vi "Get Source Directories.vi"() -> (1 "Runtime Dir":path, 2 "Protos Dir":path, 3 "Source Dir":path)   [LabVIEW 2020]
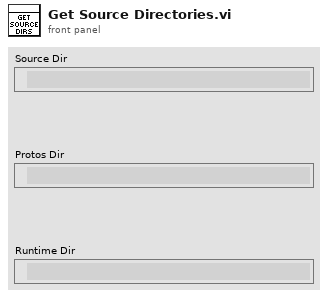
[diagram p1: front panel]
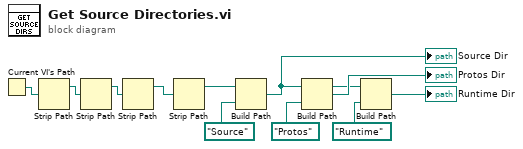
[diagram p0: block diagram]
diagram:
  n1 = Current VI's Path() -> (path=w8:path)
  n2 = Strip Path(path=w8) -> (stripped path=w9:path)  [unwired: 1 out]
  n3 = Strip Path(path=w9) -> (stripped path=w2:path)  [unwired: 1 out]
  n4 = Strip Path(path=w2) -> (stripped path=w4:path)  [unwired: 1 out]
  n5 = Strip Path(path=w4) -> (stripped path=w3:path)  [unwired: 1 out]
  n6 = Build Path(base path=w3, name or relative path=path "Source") -> (appended path=w1:path)
  "Source Dir" <- w1
  n7 = Build Path(base path=w1, name or relative path=path "Protos" ("Proto File Path")) -> (appended path=→"Protos Dir":path)
  n8 = Build Path(base path=w1, name or relative path=path "Runtime" ("Target Project")) -> (appended path=→"Runtime Dir":path)
